vi "OCU_Main.vi"() -> ()   [LabVIEW 2013]
doc: "To be executed on the Opperator Control Unit (laptop), which communicates to a variety of platforms for the sailbot boat to send missions to complete, override commands, and to monitor the status of the boat and parts of the code run on it. It should be run in parallel with \"Main.vi\" in the cRIO code foler. \n\nCreaded by Victoria Coleman and Elizabeth Mahon (03/14)"
uses:
  cRIO_Code/Data/TypeDefs/MissionTypeControl.ctl
  cRIO_Code/Data/TypeDefs/UTM Location.ctl
  cRIO_Code/Data/TypeDefs/MissionDescription.ctl
  cRIO_Code/Data/TypeDefs/MainsailPositionIndicator.ctl
  cRIO_Code/Data/TypeDefs/JibPositionIndicator.ctl
  cRIO_Code/Data/TypeDefs/Rudder Set Suggestions.ctl
  cRIO_Code/Data/TypeDefs/OverrideMode.ctl
  cRIO_Code/Data/TypeDefs/Constants for OCU Tuning.ctl
  cRIO_Code/Data/TypeDefs/MotorSetup.ctl
  cRIO_Code/Data/TypeDefs/DynamixelSetupInfo.ctl
  cRIO_Code/Logic/Classes/Missions/GenericMission/GenericMission.lvclass
  RIO-OCU_Comm/ToRIO.ctl
  CommandMessages.ctl
  Location of Think.ctl
  cRIO_Code/Logic/Classes/Missions/GoTo/GoTo.lvclass
  cRIO_Code/Logic/Classes/Missions/RoundBouy/RoundBouy.lvclass
  cRIO_Code/Logic/Classes/Missions/PassBouy/PassBouy.lvclass
  cRIO_Code/Logic/Classes/Missions/StationKeeping/StationKeeping.lvclass
  <vilib>/event_ctls.llb/eventvkey.ctl
  RIO-OCU_Comm/NetworkStreams/Writer/NetworkStreamWriter.lvclass
  RIO-OCU_Comm/NetworkStreams/Reader/NetworkStreamReader.lvclass
panel:
  in  "Do \"Initialize Me!\" Before running":enum32{"Initialize Me!", "Tuneable Constants"}(tab)
  in  "Boat Type":T1(ring)=enum."Simulation"
  in  "OCU Tuning Constants":T2
  out "Reader\nConnected?":bool
  in  "Main Tab Structure":T5(tab)
  in  "Setting Missions with Map Internal Tab":T6(tab)
  out "Robot Location":T7 {"North" format="%#_10f"; "East" format="%#_8f"}
  in  "Main":T8
  in  "Jib":T9
  in  "Rudder Setpoint":T10 min=-1.0 max=1.0 scale=1.0..-1.0
  in  "OverrideMode":T11
  out "Current Missions":T12[](array[typedef]) {"Points of Interest"."North" format="%#_10f"; "Points of Interest"."East" format="%#_8f"}
  out "# of Missions":i32
  in  "DeleteMission":bool
  in  "ID# To Delete":u16
  in  "Timeout (s)":dbl=-1.0
  in  "Duration (s)\n[For in-box mission]":dbl=-1.0
  in  "Tolerance (m)":dbl
  in  "Points of Interest":T7[](array[typedef]) {"North" format="%#_10f"; "East" format="%#_8f"}
  in  "Mission Type":T13
  in  "CreateMission":bool
  out "Error out":errorcluster
  out "Writter\nConnected?":bool
  in  "stop":bool
  # "RUN MAIN.VI FIRST. SERIOUSLY"
  # "Add a \"which boat are we\" notifier. e.g. Blackbody, Damn Yankee, Simulator, etc."
  # "If you forgot to set the boat type, you must restart the code"
  # "Reorganize\nthis section,\nmaybe split\nthe cluster\nup"
  # "PUT MAP HERE"
  # "See old OCU for commands down here. See if those are still relevant"
  # "Log Message [important that we implement this one]"
  # "Font Size"
  # "# of Waypoints"
  # "Save Image"
  # "This is where you should be able to clilck the map and set a waypoint. Look in the [Mission Map] [Mission Edit]tab in the old OCU\n(\\Software\\0-OCU\\0 Code\\0 OCU.vi)\nand check out how they set up and documented the pojnt and click operation.\nEric, 4/5/14"
  # "Add Load MDF, Save MDF, and Clear Mission functionality. Clear missions would clear all current missions. Look at old OCU for examples"
  # "Look in the [Mission Map][Monitering]tab in the old OCU\n(\\Software\\0-OCU\\0 Code\\0 OCU.vi)\nand check out how they displayed the boat information during runtime. Try and make the indicators pretty and try to give only critical information \n\nEric, 4/5/14"
  # "Look in the lower right of the old OCU\n(\\Software\\0-OCU\\0 Code\\0 OCU.vi)\nand check out how they tweaked the simulator during runtime. Do this later.\n\nEric, 4/5/14"
  # "Set wind speed"
  # "Set water current speed"
  # "Set boat position"
  # "KEY MAPPINGS TO ACTUATOR MOVEMENT:\n\n\"Up\" -- Main out    |  \"Page Down\" -- Jib out\n\"Down\" -- Main in  |  \"Right\" -- Jib in\n\n\"Page Up\" -- rudder right\n\"Left\" -- rudder left"
  # "PUT MAP HERE"
  # "Add whatever feedback would be useful here"
  # "TODO: We should convert this section so that it looks more like the \"Manual Mission Input\" section of the old OCU\n\\Software\\0-OCU\\0 Code\\0 OCU.vi"
  # "Add the \"Local GPS\" section of the old code so that we can grab GPS points from the boat and save them as waypoints or points of interest."
  # "TODO: When you delete the last mission, make idle take its place. Then when the next mission is initialized, delete the idle mission"
  # "PUT ALL THE BOAT DATA HERE\nLook at the Detailed Telemetry section of the old OCU for inspiration on how to organize information"
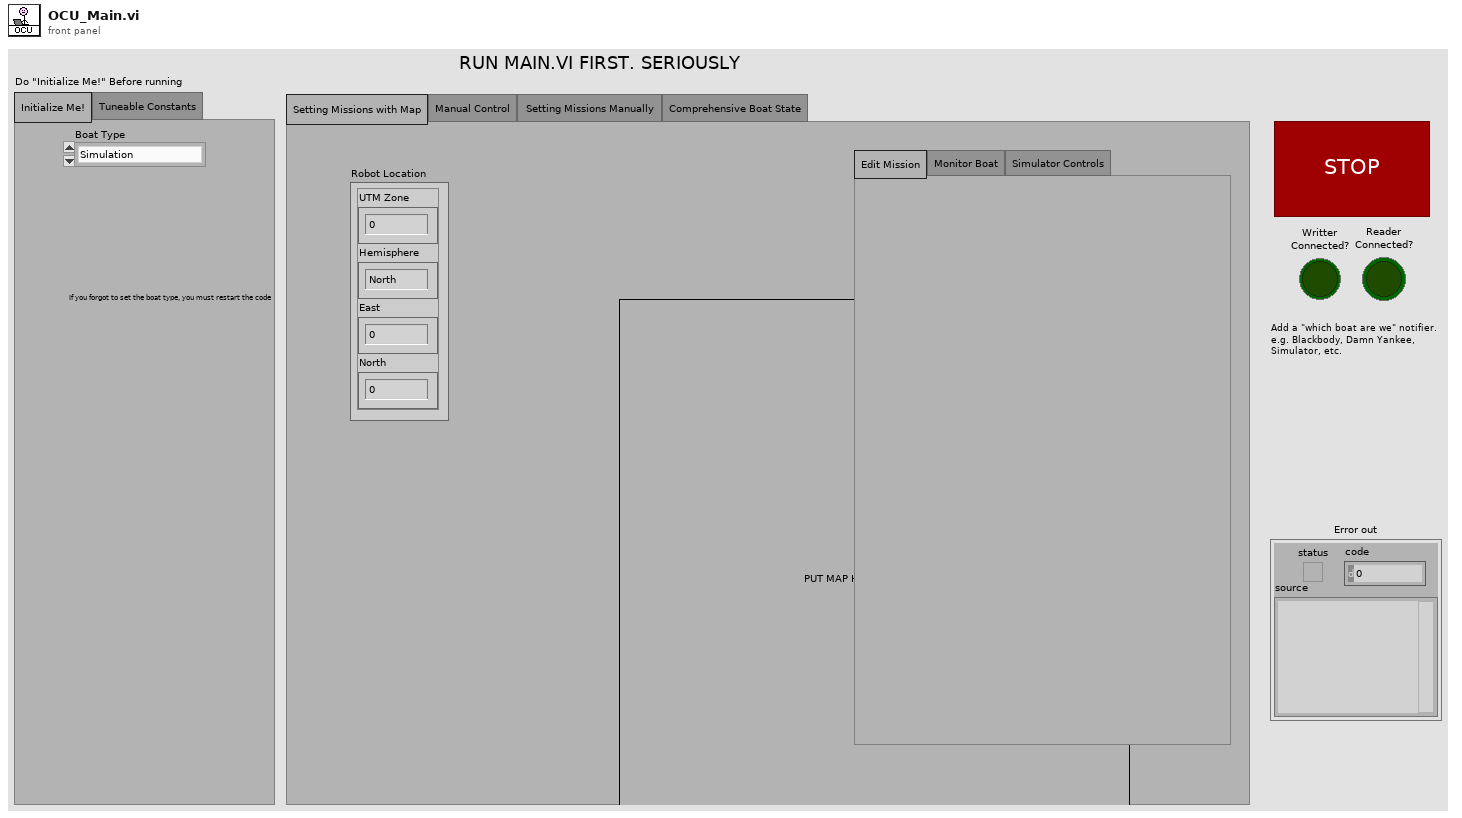
[diagram p1: front panel]
types:
  T1 = enum16{"Blackbody Radiation", "Little boats", "Simulation", "Damn Yankee"}
  T2 = typedef "Constants for OCU Tuning.ctl" = cluster{"Motor Setting Constant":T3, "Irons Range (deg)":dbl}
  T3 = typedef "MotorSetup.ctl" = cluster{"Main Dynamixel Set Data":T4, "Rudder Dynamixel Set Data":T4, "Jib Dynamixel Set Data":T4}
  T4 = typedef "DynamixelSetupInfo.ctl" = cluster{"Lower Winch Bound":dbl, "Upper Winch Bound":dbl, "Reverse Winch Direction?":bool, "Dynamixel Cycle Number":i32}
  T5 = enum32{"Setting Missions with Map", "Manual Control", "Setting Missions Manually ", "Comprehensive Boat State"}
  T6 = enum32{"Edit Mission", "Monitor Boat", "Simulator Controls"}
  T7 = typedef "UTM Location.ctl" = cluster{"UTM Zone":dbl, "Hemisphere":enum16{"North", "South"}, "East":dbl, "North":dbl}
  T8 = typedef "MainsailPositionIndicator.ctl" = dbl
  T9 = typedef "JibPositionIndicator.ctl" = dbl
  T10 = typedef "Rudder Set Suggestions.ctl" = dbl
  T11 = typedef "OverrideMode.ctl" = enum16{"None", "Rudder", "Sails", "Both"}
  T12 = typedef "MissionDescription.ctl" = cluster{"Duration (s)":dbl, "Timeout (s)":dbl, "Tolerance (m)":dbl, "Mission Type":T13, "Points of Interest":T7[], "ID#":i32}
  T13 = typedef "MissionTypeControl.ctl" = enum16{"Idle at Point", "Drive to Waypoint", "Round Buoy to Port", "Round Buoy to Starboard", "Pass Between Buoys", "Station Keeping"}
  T14 = typedef "Location of Think.ctl" = string
  T15 = typedef "CommandMessages.ctl" = enum16{"Pass", "OverrideMode", "Add mission", "Delete mission", "Change constants"}
  T16 = typedef "ToRIO.ctl" = cluster{"Commands":T15, "Variant":variant}
  T17 = typedef "eventvkey.ctl" = enum16{"ASCII", "Enter", "Return", "Shift", "Ctrl", "Alt", "Cmd", "Opt", "Caps", "NumLock", "Clear", "Break", "Up", "Down", "Left", "Right", "Insert", "Delete", "Home", "End", "PageUp", "PageDown", "Escape", "Help", "Pause", "ScrollLock", "F1", "F2", "F3", "F4", "F5", "F6", "F7", "F8", "F9", "F10", "F11", "F12", "F13", "F14", "F15", "F16", "F17", "F18", "F19", "F20", "F21", "F22", "F23", "F24", "Play", "VolumeUp", "VolumeDown", "Mute", "Two Byte Char"}
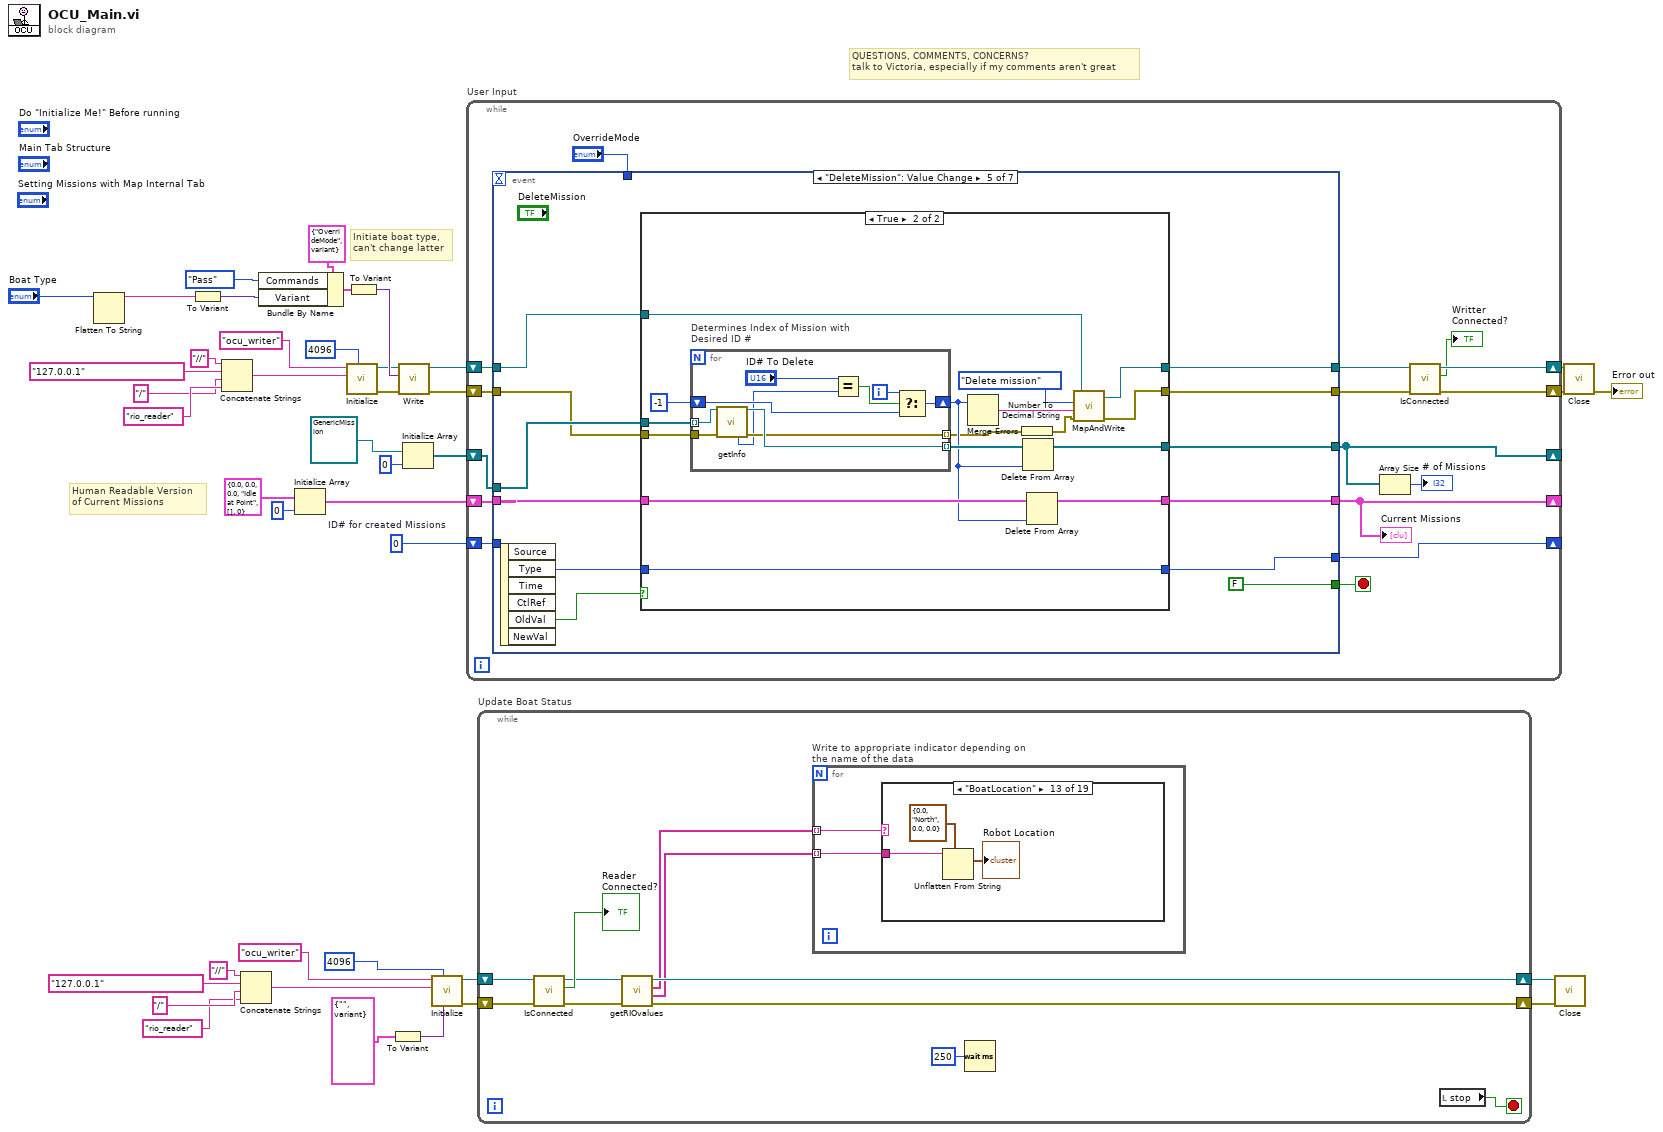
[diagram p0: block diagram]
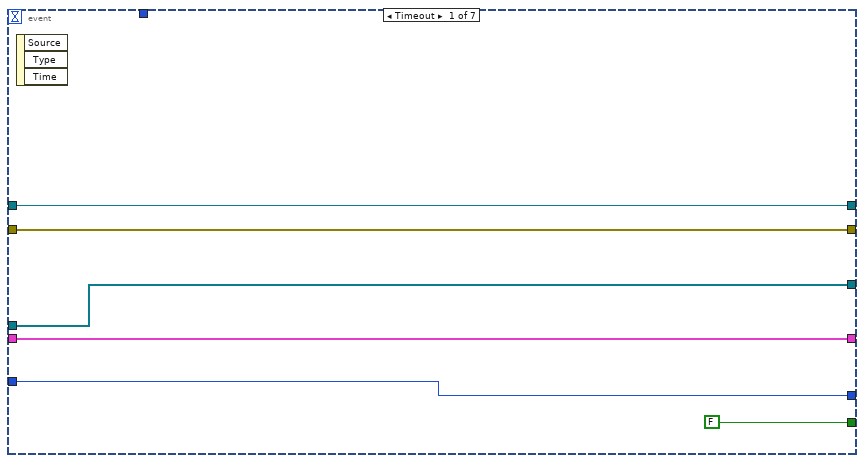
[diagram p20: hidden frame]
diagram:
  w19 = 0  # ID# for created Missions
  # "Initiate boat type,\ncan't change latter"
  # "QUESTIONS, COMMENTS, CONCERNS? \ntalk to Victoria, especially if my comments aren't great"
  # "Human Readable Version\nof Current Missions"
  n1 = Flatten To String(anything="Boat Type") -> (data string=w14:string)  [unwired: 3 in, 2 out]
  n2 = To Variant(anything=w14) -> (Variant=w17:variant)
  n3 = Concatenate Strings("//" ("string"), T14 "127.0.0.1" ("Location of THINK"), "/", "rio_reader" ("string")) -> (w32:string)
  n4 = Concatenate Strings("//" ("string"), T14 "127.0.0.1" ("Location of THINK"), "/", "rio_reader" ("string")) -> (w7:string)
  n5 = Bundle By Name(cluster=T16 {"Commands"=enum."OverrideMode", "Variant"=variant} ("To RIO"), "Commands"=CommandMessages."Pass", "Variant"=w17) -> (w16:T16)
  n6 = Initialize Array "Initialize Array"(T12 {"Duration (s)"=0.0, "Timeout (s)"=0.0, "Tolerance (m)"=0.0, "Mission Type"=enum."Idle at Point", "Points of Interest"=[], "ID#"=0} ("input cluster"), 0 ("dimension size")) -> (w37:T12[])
  n7 = call "Initialize.vi"("writer buffer size"=4096, "reader url"=w32, "writer name"="ocu_writer") -> ("error out"=w22:errorcluster, "NetworkStreamWriter out"=w23:refnum<class "NetworkStreamWriter.lvclass">)  [unwired: 7 in]
  n8 = To Variant(anything=w16) -> (Variant=w25:variant)
  n9 = To Variant(anything=cluster{"Name":string, "value":variant} {"Name"="", "value"=variant}) -> (Variant=w5:variant)
  n10 = call "Write.vi"("error in (no error)"=w22, "element"=w25, "NetworkStreamWriter in"=w23) -> ("error out"=w21:errorcluster, "NetworkStreamWriter out"=w20:refnum<class "NetworkStreamWriter.lvclass">)  [unwired: 7 in]
  n11 = Initialize Array "Initialize Array"(refnum<class "GenericMission.lvclass"> refnum ("GenericMission.lvclass"), 0 ("dimension size")) -> (w40:refnum<class "GenericMission.lvclass">[])
  n12 = call "Initialize.vi"("Default return"=w5, "reader buffer size"=4096 ("writer buffer size"), "writer url"=w7, "reader name"="ocu_writer" ("writer name")) -> ("error out"=w2:errorcluster, "NetworkStreamReader out"=w4:refnum<class "NetworkStreamReader.lvclass">)  [unwired: 6 in]
  n13 = while "User Input" {
    shift-right: [w51] -> _
    shift-left: w40 -> [w57]
    shift-right: [w55] -> _
    shift-left: w19 -> [w56]
    shift-right: [w52] -> _
    shift-left: w37 -> [w53]
    shift-right: [w44] -> w30
    shift-left: w21 -> [w49]
    shift-right: [w46] -> w31
    shift-left: w20 -> [w48]
    stop <- w50 stop-if-true
    n14 = event shown="[4] \"DeleteMission\": Value Change" {
      selector: _ -> [_ _ _ _ _ _ _]
      dyn-events: _ -> [_ _ _ _ _ _ _]
      timeout: _ -> [_ _ _ _ _ _ _]
      tunnel: w57 -> [w62 w68 w80 w123 w163 _ _]
      tunnel: [w62 w68 w79 w123 w162 _ _] -> w51
      tunnel: w56 -> [w63 w67 w81 w125 w157 _ _]
      tunnel: [w63 w67 w75 w125 w158 _ _] -> w55
      tunnel: w53 -> [w60 w66 w78 w124 w161 _ _]
      tunnel: [w60 w66 w77 w124 w160 _ _] -> w52
      tunnel: [FALSE TRUE FALSE _ FALSE _ _] -> w50
      tunnel: [w59 w65 w73 w120 w155 w197 w204] -> w45
      tunnel: w48 -> [w58 w64 w72 w126 w153 w198 w206]
      tunnel: w49 -> [w59 w65 w71 w121 w154 w199 w207]
      tunnel: [w58 w64 w70 w122 w152 w196 w205] -> w47
      tunnel: "OverrideMode" -> [_ _ _ w115 _ _ w203]
      event Timeout {
        n15 = event-data() -> ()  [unwired: 1 in, 3 out]
      }
      event "stop": Value Change {
        n16 = event-data() -> ()  [unwired: 1 in, 6 out]
      }
      event "CreateMission": Value Change {
        n17 = event-data() -> ("OldVal"=w74:bool)  [unwired: 1 in, 5 out]
        n18 = case shown="True" w74 {
          tunnel: w81 -> [w84 w94]
          tunnel: w80 -> [w86 w107]
          tunnel: [w86 w106] -> w79
          tunnel: w78 -> [w85 w103]
          tunnel: [w85 w102] -> w77
          tunnel: [w84 w97] -> w75
          tunnel: [w83 w87] -> w73
          tunnel: w72 -> [w82 w91]
          tunnel: w71 -> [w83 w96]
          tunnel: [w82 w88] -> w70
          frame False {
          }
          frame True {
            # "Init. mission\nObject"
            # "send created\nmessage to\nForebrain"
            # "Converts to human-\nreadable form, stores\nlocal array"
            n19 = case shown="\"Idle at Point\", Default" "Mission Type" {
              tunnel: [w109 w110 w111 w112 w113 w114] -> w108
              frame "Idle at Point", Default {
                w109 = refnum<class "GoTo.lvclass"> refnum  # GoTo.lvclass
              }
              frame "Drive to Waypoint" {
                w110 = refnum<class "GoTo.lvclass"> refnum  # GoTo.lvclass
              }
              frame "Round Buoy to Port" {
                w111 = refnum<class "RoundBouy.lvclass"> refnum  # RoundBouy.lvclass
              }
              frame "Round Buoy to Starboard" {
                w112 = refnum<class "RoundBouy.lvclass"> refnum  # RoundBouy.lvclass
              }
              frame "Pass Between Buoys" {
                w113 = refnum<class "PassBouy.lvclass"> refnum  # PassBouy.lvclass
              }
              frame "Station Keeping" {
                w114 = refnum<class "StationKeeping.lvclass"> refnum  # StationKeeping.lvclass
              }
            }
            n20 = call-dynamic "InitializeMission.vi"("GenericMission in"=w108, "Duration (s)"="Duration (s)\n[For in-box mission]", "Mission Type"="Mission Type", "ID#"=w94, "Points of Interest"="Points of Interest", "Error In"=w96, "Timeout (s)"="Timeout (s)", "Tolerance (m)"="Tolerance (m)") -> ("GenericMission out"=w95:refnum<class "GenericMission.lvclass">)  [unwired: 6 in, 1 out]
            n21 = Bundle By Name(cluster=T12 {"Duration (s)"=0.0, "Timeout (s)"=0.0, "Tolerance (m)"=0.0, "Mission Type"=enum."Idle at Point", "Points of Interest"=[], "ID#"=0} ("input cluster"), "Duration (s)"="Duration (s)\n[For in-box mission]", "Points of Interest"="Points of Interest", "Timeout (s)"="Timeout (s)", "Tolerance (m)"="Tolerance (m)", "Mission Type"="Mission Type", "ID#"=w94) -> (w104:T12)
            n22 = Flatten To String(anything=w95) -> (data string=w90:string, error out=w89:errorcluster)  [unwired: 3 in, 1 out]
            n23 = call "MapAndWrite.vi"("error in (no error)"=w89, "String_Cast_of_Info"=w90, "Commands"=CommandMessages."Add mission", "NetworkStreamWriter in"=w91) -> ("error out"=w87:errorcluster, "NetworkStreamWriter out"=w88:refnum<class "NetworkStreamWriter.lvclass">)  [unwired: 2 in]
            n24 = Insert Into Array(array=w103, new element=w104) -> (w102:T12[])  [unwired: 1 in]
            n25 = Increment(x=w94) -> (x+1=w97:i32)
            n26 = Insert Into Array(array=w107, new element=w95) -> (w106:refnum<class "GenericMission.lvclass">[])  [unwired: 1 in]
          }
        }
      }
      event Key Down; Key Repeat {
        n27 = event-data() -> ("VKey"=w116:T17)  [unwired: 1 in, 9 out]
        n28 = case "Only if Special key pressed" shown="Default" w116 {
          selector: w116 -> [_ w134]
          tunnel: w126 -> [w128 w130]
          tunnel: [w128 w131] -> w122
          tunnel: w121 -> [w127 w133]
          tunnel: [w127 w132] -> w120
          tunnel: "Rudder Setpoint" -> [_ w137]
          tunnel: "Jib" -> [_ w136]
          tunnel: "Main" -> [_ w135]
          tunnel: w115 -> [_ w129]
          frame "ASCII" {
            # "No special key pressed :("
          }
          frame Default {
            n29 = case "Only executes of any actuators are in override mode" shown="Default" w129 {
              selector: w129 -> [_ w144]
              tunnel: w137 -> [_ w149]
              tunnel: w136 -> [_ w150]
              tunnel: w135 -> [_ w151]
              tunnel: w134 -> [_ w147]
              tunnel: w133 -> [w139 w146]
              tunnel: [w139 w148] -> w132
              tunnel: [w138 w143] -> w131
              tunnel: w130 -> [w138 w145]
              frame "None" {
              }
              frame Default {
                # "KEY MAPPINGS TO ACTUATOR MOVEMENT:\n\"Page Up\" -- rudder right       |    \"Up\" -- Main out          |     \"Page Down\" -- Jib out\n\"Left\" -- rudder left                  |      \"Down\" -- Main in     |      \"Right\" -- Jib in"
                n30 = call "Write_NetworkStream_OCU_Override.vi"("VKey"=w147, "NetworkStreamWriter in"=w145, "Mainsail Position"=w151, "Jib Position"=w150, "Rudder Setpoint"=w149, "error in (no error)"=w146, "OverrideMode"=w144) -> ("NetworkStreamWriter out"=w143:refnum<class "NetworkStreamWriter.lvclass">, "Main Position"=w142:T8, "Jib Position"=w141:T9, "Rudder Position"=w140:T10, "error out"=w148:errorcluster)  [unwired: 4 in]
                n31 = local write "Main"(w142) -> ()
                n32 = local write "Rudder Setpoint"(w140) -> ()
                n33 = local write "Jib"(w141) -> ()
              }
            }
          }
        }
      }
      event "DeleteMission": Value Change {
        n34 = event-data() -> ("OldVal"=w156:bool)  [unwired: 1 in, 5 out]
        n35 = case shown="True" w156 {
          tunnel: w163 -> [w168 w184]
          tunnel: [w168 w172] -> w162
          tunnel: w161 -> [w167 w181]
          tunnel: [w167 w180] -> w160
          tunnel: [w166 w179] -> w158
          tunnel: w157 -> [w166 w179]
          tunnel: [w165 w170] -> w155
          tunnel: w154 -> [w165 w177]
          tunnel: w153 -> [w164 w176]
          tunnel: [w164 w169] -> w152
          frame False {
          }
          frame True {
            n36 = for "Determines Index of Mission with\nDesired ID #" {
              tunnel: w184 -> [w194] mode=indexing
              tunnel: [w193] -> w182 mode=indexing
              shift-right: [w190] -> w178
              shift-left: -1 -> [w189]
              tunnel: [w188] -> w173 mode=indexing
              tunnel: w177 -> [w187]
              i -> [w191]
              n37 = call-dynamic "getInfo.vi"("GenericMission in"=w194, "error in (no error)"=w187) -> ("GenericMission out"=w193:refnum<class "GenericMission.lvclass">, "ID#"=w185:u16, "error out"=w188:errorcluster)  [unwired: 5 in, 6 out]
              n38 = Equal?(x="ID# To Delete", y=w185) -> (x = y?=w192:bool)
              n39 = Select(t=w191, s=w192, f=w189) -> (s? t:f=w190:i32)
            }
            n40 = Number To Decimal String(number=w178) -> (decimal integer string=w174:string)  [unwired: 1 in]
            n41 = Merge Errors(w173) -> (w171:errorcluster)
            n42 = Delete From Array(array=w182, index=w178) -> (array with subset deleted=w172:refnum<class "GenericMission.lvclass">[])  [unwired: 1 in, 1 out]
            n43 = Delete From Array(array=w181, index=w178) -> (array with subset deleted=w180:T12[])  [unwired: 1 in, 1 out]
            n44 = call "MapAndWrite.vi"("error in (no error)"=w171, "String_Cast_of_Info"=w174, "Commands"=CommandMessages."Delete mission", "NetworkStreamWriter in"=w176) -> ("error out"=w170:errorcluster, "NetworkStreamWriter out"=w169:refnum<class "NetworkStreamWriter.lvclass">)  [unwired: 2 in]
          }
        }
      }
      event Value Change {
        n45 = event-data() -> ()  [unwired: 1 in, 6 out]
        n46 = Flatten To String(anything="OCU Tuning Constants", error in (no error)=w199) -> (data string=w201:string, error out=w200:errorcluster)  [unwired: 2 in, 1 out]
        n47 = call "MapAndWrite.vi"("error in (no error)"=w200, "String_Cast_of_Info"=w201, "Commands"=CommandMessages."Change constants", "NetworkStreamWriter in"=w198) -> ("error out"=w197:errorcluster, "NetworkStreamWriter out"=w196:refnum<class "NetworkStreamWriter.lvclass">)  [unwired: 2 in]
      }
      event Value Change {
        # "Just an obscure key\nto make everything update\n(hackish solution to reuse\nvi)"
        n48 = event-data() -> ()  [unwired: 1 in, 6 out]
        n49 = local read "Main Tab Structure"() -> (w209:T5)
        n50 = local read "Main"() -> (w211:T8)
        n51 = local read "Jib"() -> (w210:T9)
        n52 = call "Write_NetworkStream_OCU_Override.vi"("VKey"=eventvkey."F24", "NetworkStreamWriter in"=w206, "Mainsail Position"=w211, "Jib Position"=w210, "Rudder Setpoint"=w209, "error in (no error)"=w207, "OverrideMode"=w203) -> ("NetworkStreamWriter out"=w205:refnum<class "NetworkStreamWriter.lvclass">, "error out"=w204:errorcluster)  [unwired: 4 in, 3 out]
      }
    }
    "Current Missions" <- w52
    n53 = Array Size(array=w51) -> (size(s)=→"# of Missions":i32)
    n54 = call "IsConnected.vi"("error in (no error)"=w45, "NetworkStreamWriter in"=w47) -> ("error out"=w44:errorcluster, "Connected?"=→"Writter\nConnected?":bool, "NetworkStreamWriter out"=w46:refnum<class "NetworkStreamWriter.lvclass">)  [unwired: 7 in]
  }
  n55 = while "Update Boat Status" {
    shift-right: [w217] -> w3
    shift-left: w4 -> [w221]
    shift-right: [w212] -> w1
    shift-left: w2 -> [w220]
    stop <- w222 stop-if-true
    n56 = call "IsConnected.vi"("error in (no error)"=w220, "NetworkStreamReader in"=w221) -> ("error out"=w216:errorcluster, "Connected?"=→"Reader\nConnected?":bool, "NetworkStreamReader out"=w218:refnum<class "NetworkStreamReader.lvclass">)  [unwired: 7 in]
    n57 = call "getRIOvalues.vi"("error in (no error)"=w216, "NetworkStreamReader in"=w218) -> ("error out"=w212:errorcluster, "data"=w213:string[], "names"=w214:string[], "NetworkStreamReader out"=w217:refnum<class "NetworkStreamReader.lvclass">)  [unwired: 6 in]
    n58 = for "Write to appropriate indicator depending on the name of the data" {
      tunnel: w214 -> [w224] mode=indexing
      tunnel: w213 -> [w223] mode=indexing
      n59 = case shown="\"BoatLocation\"" w224 {
        tunnel: w223 -> [_ _ _ _ _ _ _ _ _ _ _ _ w227 _ _ _ _ _ _]
        frame Default {
          # "unknown name"
        }
        frame "BoatSpeed" {
        }
        frame "WindSpeed" {
        }
        frame "SailPositions" {
        }
        frame "MissionCheckOff" {
        }
        frame "SpeedOverWater" {
        }
        frame "BoatDirection" {
        }
        frame "RudderPosition" {
        }
        frame "Luffing" {
        }
        frame "RudderForce" {
        }
        frame "BatteryVoltage" {
        }
        frame "StayForces" {
        }
        frame "BoatLocation" {
          n60 = Unflatten From String(type=T7 {"UTM Zone"=0.0, "Hemisphere"=enum."North", "East"=0.0, "North"=0.0} ("UTM Location"), binary string=w227) -> (value=→"Robot Location":T7)  [unwired: 3 in, 2 out]
        }
        frame "Pitch" {
        }
        frame "Roll" {
        }
        frame "RateOfTurn" {
        }
        frame "RelWindDirection" {
        }
        frame "AbsWindDirection" {
        }
        frame "DynamixelTorques" {
        }
      }
    }
    n61 = Wait (ms)(milliseconds to wait=u32 250) -> ()  [unwired: 1 out]
    n62 = local read "stop"() -> (w222:bool)
  }
  n63 = call "Close.vi"("error in (no error)"=w1, "NetworkStreamReader in"=w3) -> ()  [unwired: 9 in, 1 out]
  n64 = call "Close.vi"("error in (no error)"=w30, "NetworkStreamWriter in"=w31) -> ("error out"=→"Error out":errorcluster)  [unwired: 9 in]
